vi "ProcessOldFilesOnTarget.vi"   [LabVIEW 2014]
uses:
  IndoorData_class/IndoorData.lvclass
  <vilib>/MakerHub/Toolbox/LMH-Toolbox.lvlib
types:
  T1 = enum16{"open", "replace", "create", "open or create", "replace or create", "replace or create with confirmation"}
  T2 = typedef "IndoorData.lvclass/BufferedReadings.ctl" = cluster{"Time":dbl[], "Temp":dbl[], "RH":dbl[]}
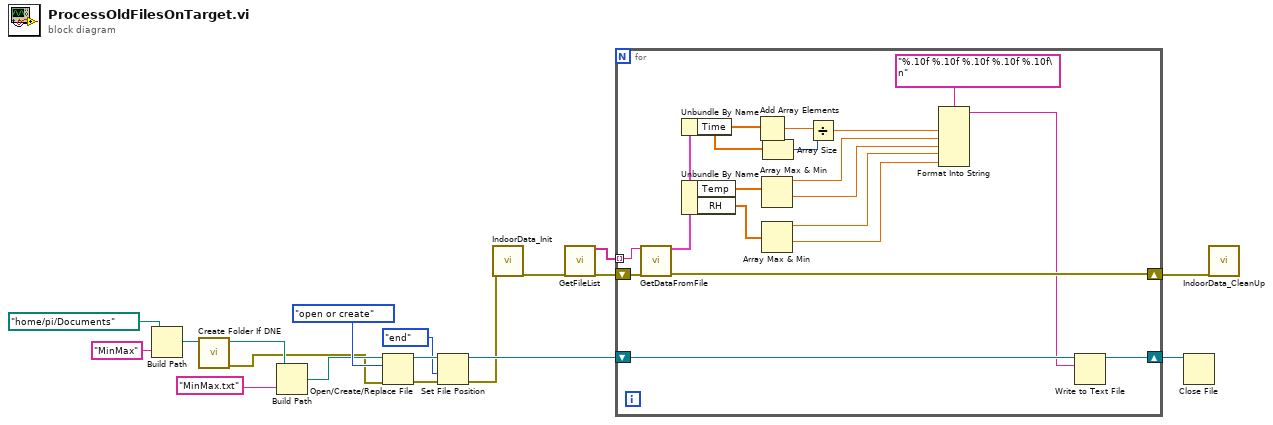
[diagram p0: block diagram]
diagram:
  n1 = Build Path(base path=path "/home/pi/Documents", name or relative path="MinMax") -> (appended path=w8:path)
  n2 = call <vilib>:"Create Folder If DNE.vi"("Folder Path"=w8) -> ("Error Out"=w2:errorcluster, "Dup Path"=w7:path)  [unwired: 9 in]
  n3 = Build Path(base path=w7, name or relative path="MinMax.txt") -> (appended path=w5:path)
  n4 = Open/Create/Replace File(file path (use dialog)=w5, error in=w2, operation (0:open)=T1."open or create") -> (refnum out=w14:refnum<file>, error out=w3:errorcluster)  [unwired: 3 in, 1 out]
  n5 = Set File Position(refnum=w14, from (0:start)=enum16{"start", "end", "current"}."end", error in=w3) -> (refnum out=w12:refnum<file>, error out=w1:errorcluster)  [unwired: 1 in]
  n6 = call "IndoorData_Init.vi"("error in (no error)"=w1) -> ("error out"=w16:errorcluster)  [unwired: 17 in, 1 out]
  n7 = call "GetFileList.vi"("error in (no error)"=w16) -> ("filenames"=w17:string[], "error out"=w18:errorcluster)  [unwired: 17 in]
  n8 = for {
    shift-right: [w36] -> w4
    shift-left: w18 -> [w35]
    tunnel: w17 -> [w34] mode=indexing
    shift-right: [w20] -> w11
    shift-left: w12 -> [w21]
    n9 = call "GetDataFromFile.vi"("FileName"=w34, "error in (no error)"=w35) -> ("FileData"=w33:T2, "error out"=w36:errorcluster)  [unwired: 16 in]
    n10 = Unbundle By Name(w33) -> ("Time"=w30:dbl[])
    n11 = Unbundle By Name(w33) -> ("Temp"=w31:dbl[], "RH"=w32:dbl[])
    n12 = Add Array Elements(numeric array=w30) -> (sum=w29:dbl)
    n13 = Array Max & Min(array=w31) -> (max value=w25:dbl, min value=w24:dbl)  [unwired: 2 out]
    n14 = Array Max & Min(array=w32) -> (max value=w23:dbl, min value=w22:dbl)  [unwired: 2 out]
    n15 = Array Size(array=w30) -> (size(s)=w28:i32)
    n16 = Divide(x=w29, y=w28) -> (x/y=w26:dbl)
    n17 = Format Into String(format string="%.10f %.10f %.10f %.10f %.10f\n", w26, w25, w24, w23, w22) -> (resulting string=w19:string)  [unwired: 2 in, 1 out]
    n18 = Write to Text File(file (use dialog)=w21, text=w19) -> (refnum out=w20:refnum<file>)  [unwired: 2 in, 2 out]
  }
  n19 = Close File(refnum=w11) -> ()  [unwired: 1 in, 2 out]
  n20 = call "IndoorData_CleanUp.vi"("error in (no error)"=w4) -> ()  [unwired: 18 in, 1 out]
